vi "CalculateBoundingBox.vi"(8 "error in (no error)":errorcluster, 11 "Items":refnum<vi>[](array[refnum])) -> (0 "error out":errorcluster, 1 "Current bounding box position":cluster{"Left":i32, "Top":i32}, 2 "Size of bounding box for items":T1, 3 "Items out (dup)":refnum<vi>[](array[refnum]))   [LabVIEW 2017, in "ErrorStructureDrawer.lvlib"]
doc: "Calculate the height and width of a bounding box that would contain the specified items."
uses:
  <vilib>/Utility/miscctls.llb/LVBoundsTypeDef.ctl
  ErrorStructureDrawer.lvlib
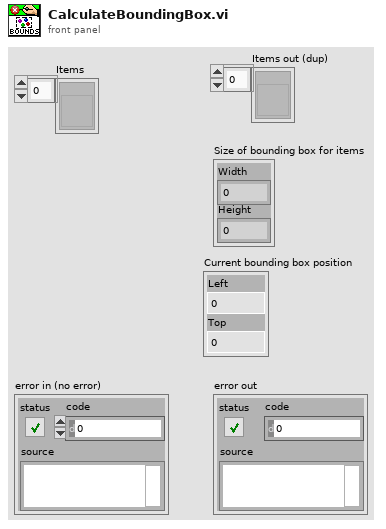
[diagram p1: front panel]
types:
  T1 = typedef "LVBoundsTypeDef.ctl" = cluster{"Width":u32, "Height":u32}
  T2 = typedef "LVRectTypeDef.ctl" = cluster{"Left":i16, "Top":i16, "Right":i16, "Bottom":i16}
  T3 = cluster{"Left":i32, "Top":i32, "Right":i32, "Bottom":i32}
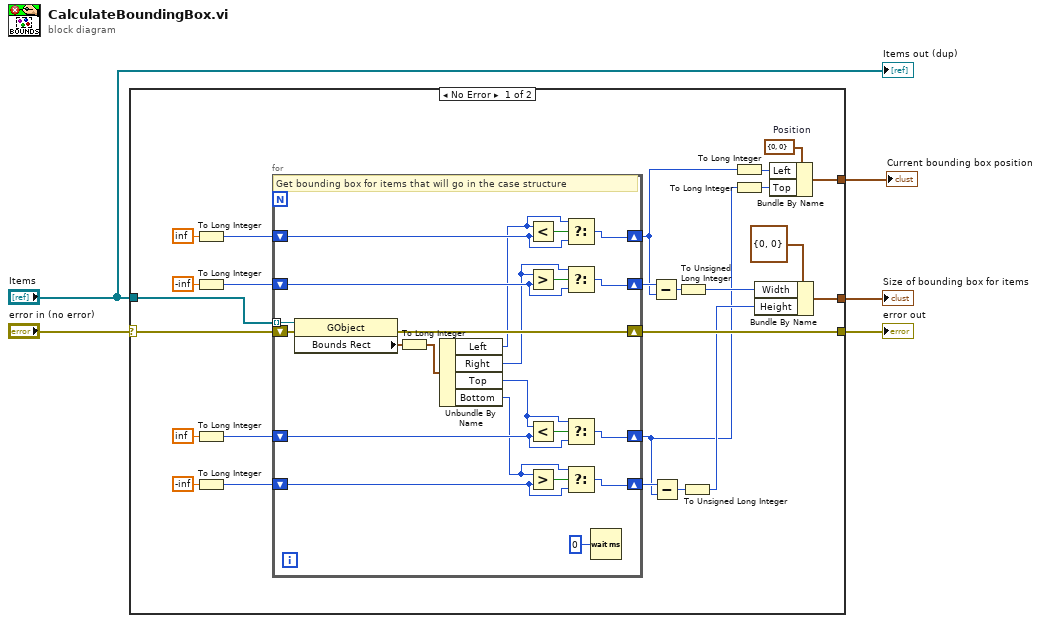
[diagram p0: block diagram]
diagram:
  n1 = case shown="No Error" "error in (no error)" {
    selector: "error in (no error)" -> [w12 w53]
    tunnel: [w30 w53] -> w5
    tunnel: [w29 _] -> w4
    tunnel: "Items" -> [w13 _]
    tunnel: [w6 _] -> w1
    frame No Error {
      w11 = cluster{"Left":i32, "Top":i32} {"Left"=0, "Top"=0}  # Position
      n2 = To Long Integer(number=inf) -> (32bit integer=w16:i32)
      n3 = To Long Integer(number=-inf) -> (32bit integer=w17:i32)
      n4 = To Long Integer(number=inf) -> (32bit integer=w19:i32)
      n5 = To Long Integer(number=-inf) -> (32bit integer=w18:i32)
      n6 = for {
        tunnel: w13 -> [w38] mode=indexing
        shift-right: [w51] -> w10
        shift-left: w16 -> [w50]
        shift-right: [w48] -> w23
        shift-left: w17 -> [w49]
        shift-right: [w42] -> w7
        shift-left: w19 -> [w43]
        shift-right: [w45] -> w24
        shift-left: w18 -> [w44]
        shift-right: [w39] -> w30
        shift-left: w12 -> [w40]
        # "Get bounding box for items that will go in the case structure"
        n7 = property class="GObject"(reference=w38, error in=w40) -> (error out=w39:errorcluster, "Bounds Rect"=w33:T2)  [unwired: 1 out]
        n8 = To Long Integer(number=w33) -> (32bit integer=w32:T3)
        n9 = Unbundle By Name(w32) -> ("Left"=w37:i32, "Right"=w36:i32, "Top"=w35:i32, "Bottom"=w34:i32)
        n10 = Less?(x=w37, y=w50) -> (x < y?=w52:bool)
        n11 = Greater?(x=w36, y=w49) -> (0:w47:bool)
        n12 = Less?(x=w35, y=w43) -> (x < y?=w41:bool)
        n13 = Greater?(x=w34, y=w44) -> (0:w46:bool)
        n14 = Select(t=w37, s=w52, f=w50) -> (s? t:f=w51:i32)
        n15 = Select(t=w36, s=w47, f=w49) -> (s? t:f=w48:i32)
        n16 = Select(t=w35, s=w41, f=w43) -> (s? t:f=w42:i32)
        n17 = Select(t=w34, s=w46, f=w44) -> (s? t:f=w45:i32)
        n18 = Wait (ms)(milliseconds to wait=u32 0) -> ()  [unwired: 1 out]
      }
      n19 = Subtract(x=w23, y=w10) -> (x-y=w25:i32)
      n20 = Subtract(x=w24, y=w7) -> (x-y=w26:i32)
      n21 = To Unsigned Long Integer(number=w25) -> (unsigned 32bit integer=w28:u32)
      n22 = To Unsigned Long Integer(number=w26) -> (unsigned 32bit integer=w27:u32)
      n23 = To Long Integer(number=w10) -> (32bit integer=w9:i32)
      n24 = To Long Integer(number=w7) -> (32bit integer=w8:i32)
      n25 = Bundle By Name(cluster=T1 {"Width"=0, "Height"=0} ("bounds"), "Width"=w28, "Height"=w27) -> (w29:T1)
      n26 = Bundle By Name(cluster=w11, "Left"=w9, "Top"=w8) -> (w6:cluster{"Left":i32, "Top":i32})
    }
    frame Error {
    }
  }
  "error out" <- w5
  "Size of bounding box for items" <- w4
  "Current bounding box position" <- w1
  "Items out (dup)" <- "Items"
